vi "KE2410_Test.vi"(8 "error in (no error)":errorcluster, 11 "KE2410 in":refnum<class "KE2410.lvclass">) -> (0 "error out":errorcluster, 3 "KE2410 out":refnum<class "KE2410.lvclass">)   [LabVIEW 2019, in "KE2410.lvclass"]
uses:
  KE2410.lvclass
  <vilib>/Platform/TimedLoop/XDataNode/timing_clust.ctl
  <vilib>/Platform/TimedLoop/XDataNode/nitl_modes.ctl
  <vilib>/Platform/TimedLoop/XDataNode/wakeup.ctl
  InstrumentSetup.vi
  <vilib>/platform/TimedLoop/XDataNode/XDataNode.xnode
  <vilib>/Platform/TimedLoop/XDataNode/XDNodeRunTimeDep.lvlib
  InstrControl.lvclass
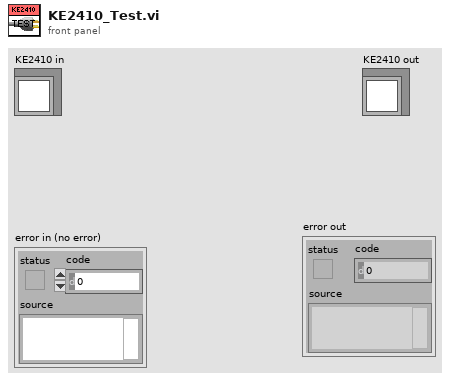
[diagram p1: front panel]
types:
  T1 = cluster{"KE 2410":cluster{"Instrument name":string, "address":refnum<visa-resource-name>, "Instrument type":u16}, "KE 6517":cluster{"Instrument name":string, "address":refnum<visa-resource-name>, "Instrument type":u16}, "KE 487":cluster{"Instrument name":string, "address":refnum<visa-resource-name>, "Instrument type":u16}, "KE 236":cluster{"Instrument name":string, "address":refnum<visa-resource-name>, "Instrument type":u16}, "WK 6440B":cluster{"Instrument name":string, "address":refnum<visa-resource-name>, "Instrument type":u16}, "WK 6425":cluster{"Instrument name":string, "address":refnum<visa-resource-name>, "Instrument type":u16}, "Pickering Matrix":cluster{"Instrument name":string, "address":refnum<visa-resource-name>, "Instrument type":u16}, "KE 2000":cluster{"Instrument name":string, "address":refnum<visa-resource-name>, "Instrument type":u16}, "KE3706A Switching":cluster{"Instrument name":string, "address":refnum<visa-resource-name>, "Instrument type":u16}, "KE 2657A":cluster{"Instrument name":string, "address":refnum<visa-resource-name>, "Instrument type":u16}, "R_METAL KE2410":cluster{"Instrument name":string, "address":refnum<visa-resource-name>, "Instrument type":u16}}
  T2 = cluster{"Current Limit":sgl, "KE2410":refnum<class "KE2410.lvclass">}
  T3 = typedef "XDNodeRunTimeDep.lvlib/timing_clust.ctl" = cluster{"Expected End [f-1]":u64, "Actual End [f-1]":u64, "Finished Late? [f-1]":bool, "Expected End [i-1]":u64, "Actual End [i-1]":u64, "Finished Late? [i-1]":bool, "Expected Start [i]":u64, "Actual Start [i]":u64, "Expected Start [f]":u64, "Actual Start [f]":u64, "Source Name":string, "Structure Name":string, "Period":i64, "Deadline":i64, "Offset":i64, "Start":i64, "Priority":i32, "Timeout":i32, "Mode":T4, "Wakeup Reason":T5, "Error":errorcluster, "Source Type":string, "Secondary Source Type":string, "Global End Time":u64, "Global Start Time":u64, "Frame Duration":u64, "Iteration Duration":u64, "Assigned CPU":i32, "I/O Scan Engine Mode":u32}
  T4 = typedef "XDNodeRunTimeDep.lvlib/nitl_modes.ctl" = enum32{"No Change", "Process missed periods, maintain original phase", "Discard missed periods, maintain original phase", "Process missed periods, ignore original phase", "Discard missed periods, ignore original phase"}
  T5 = typedef "XDNodeRunTimeDep.lvlib/wakeup.ctl" = enum32{"Normal", "Aborted", "Asynchronous wakeup", "Timing source error", "Timed loop error", "Timeout"}
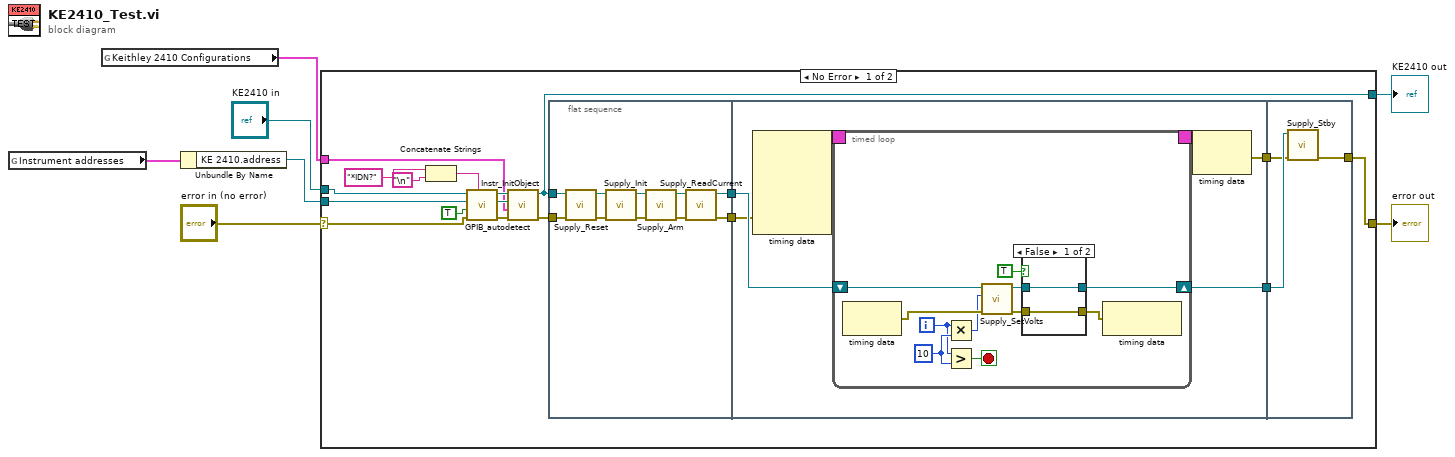
[diagram p0: block diagram]
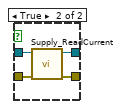
[diagram p2: hidden frame]
diagram:
  n1 = global read "InstrumentSetup.vi" "Instrument addresses"() -> (w3:T1)
  n2 = global read "InstrumentSetup.vi" "Keithley 2410 Configurations"() -> (w1:T2)
  n3 = Unbundle By Name(w3) -> ("KE 2410.address"=w2:refnum<visa-resource-name>)
  n4 = case shown="No Error" "error in (no error)" {
    selector: "error in (no error)" -> [w18 w73]
    tunnel: "KE2410 in" -> [w15 w72]
    tunnel: [w21 w72] -> w6
    tunnel: [w20 w73] -> w5
    tunnel: w2 -> [w16 _]
    tunnel: w1 -> [w12 _]
    frame No Error {
      n5 = Concatenate Strings("*IDN?" ("regular expression"), "\n") -> (w8:string)
      n6 = call-dynamic "GPIB_autodetect.vi"("ID command"=w8, "error in (no error)"=w18, "Verify GPIB address"=TRUE, "Instrument address in"=w16, "InstrControl in"=w15) -> ("error out"=w17:errorcluster, "Instrument address out"=w13:refnum<visa-resource-name>, "InstrControl out"=w14:refnum<class "KE2410.lvclass">)  [unwired: 4 in]
      n7 = call-dynamic "Instr_InitObject.vi"("error in (no error)"=w17, "Instrument Configuration"=w12, "Instrument address"=w13, "KE2410 in"=w14) -> ("error out"=w22:errorcluster, "KE2410 out"=w21:refnum<class "KE2410.lvclass">)  [unwired: 6 in]
      n8 = flat-sequence {
        tunnel: w22 -> [w30]
        tunnel: w21 -> [w29]
        tunnel: [w27] -> w25
        tunnel: [w26] -> w19
        tunnel: w25 -> [w41]
        tunnel: [w40] -> w24
        tunnel: [w37] -> w23
        tunnel: w19 -> [w36]
        tunnel: [w69] -> w20
        tunnel: w24 -> [w70]
        tunnel: w23 -> [w71]
        frame #0 {
          n9 = call-dynamic "Supply_Reset.vi"("error in (no error)"=w30, "SupplyControl in"=w29) -> ("error out"=w34:errorcluster, "SupplyControl out"=w28:refnum<class "KE2410.lvclass">)  [unwired: 8 in]
          n10 = call-dynamic "Supply_Init.vi"("error in (no error)"=w34, "SupplyControl in"=w28) -> ("error out"=w33:errorcluster, "SupplyControl out"=w35:refnum<class "KE2410.lvclass">)  [unwired: 8 in]
          n11 = call-dynamic "Supply_Arm.vi"("error in (no error)"=w33, "SupplyControl in"=w35) -> ("error out"=w31:errorcluster, "SupplyControl out"=w32:refnum<class "KE2410.lvclass">)  [unwired: 8 in]
          n12 = call-dynamic "Supply_ReadCurrent.vi"("error in (no error)"=w31, "SupplyControl in"=w32) -> ("error out"=w26:errorcluster, "SupplyControl out"=w27:refnum<class "KE2410.lvclass">)  [unwired: 7 in, 1 out]
        }
        frame #1 {
          n13 = node-c288(w36) -> (w39:T3)  [unwired: 4 in]
          n14 = timed-loop {
            timing: w39 -> [_]
            timing-out: [_] -> w38
            shift-right: [w44] -> w37
            shift-left: w41 -> [w50]
            i -> [w48]
            stop <- w47 stop-if-true
            w49 = 10
            n15 = node-c288() -> (w52:errorcluster)  [unwired: 1 in]
            n16 = Multiply(x=w48, y=w49) -> (x*y=w51:i32)
            n17 = Greater?(x=w48, y=w49) -> (0:w47:bool)
            n18 = call-dynamic "Supply_SetVolts.vi"("error in (no error)"=w52, "Volts IN [V]"=w51, "KE2410 in"=w50) -> ("error out"=w46:errorcluster, "KE2410 out"=w45:refnum<class "KE2410.lvclass">)  [unwired: 6 in, 1 out]
            n19 = case shown="False" TRUE {
              tunnel: w46 -> [w54 w58]
              tunnel: w45 -> [w53 w57]
              tunnel: [w53 w56] -> w44
              tunnel: [w54 w55] -> w43
              frame False {
              }
              frame True {
                n20 = call-dynamic "Supply_ReadCurrent.vi"("error in (no error)"=w58, "SupplyControl in"=w57) -> ("error out"=w55:errorcluster, "SupplyControl out"=w56:refnum<class "KE2410.lvclass">)  [unwired: 7 in, 1 out]
              }
            }
            n21 = node-c288(w43) -> ()  [unwired: 1 out]
          }
          n22 = node-c288(w38) -> (w40:errorcluster)
        }
        frame #2 {
          n23 = call-dynamic "Supply_Stby.vi"("error in (no error)"=w70, "SupplyControl in"=w71) -> ("error out"=w69:errorcluster)  [unwired: 8 in, 1 out]
        }
      }
    }
    frame Error {
    }
  }
  "error out" <- w5
  "KE2410 out" <- w6
